vi "Continuous Convolution (FIR).vi"   [LabVIEW 2020, in "NI_MAPro.lvlib"]
doc: "Convolves single or multiple waveforms and one or more kernels with state, allowing subsequent calls to be processed in a continuous manner. If you are convolving multiple waveforms, the VI maintains separate convolution states for each waveform."
uses:
  NI_MAPro.lvlib
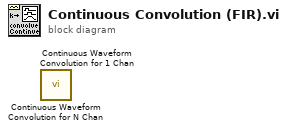
[diagram p0: block diagram]
diagram:
  n1 = call "Continuous Waveform Convolution for N Chan.vi"() -> ()  [unwired: 10 in, 2 out]
  n2 = call "Continuous Waveform Convolution for 1 Chan.vi"() -> ()  [unwired: 10 in, 2 out]
